vi "create_request_and_send.vi"(8 "error in":errorcluster, 11 "obj in":refnum<class "RequestBuilder.lvclass">) -> (0 "error out":errorcluster, 2 "request":refnum<class "Request.lvclass">, 3 "obj out":refnum<class "RequestBuilder.lvclass">)   [LabVIEW 2020, in "reqwest.lvlib" / "RequestBuilder.lvclass"]
uses:
  RequestBuilder.lvclass
  Request/Request.lvclass
  Request/request_id.ctl
  RequestBuilder.lvclass/RequestBuilder.ctl
  lv_reqwest_32.dll
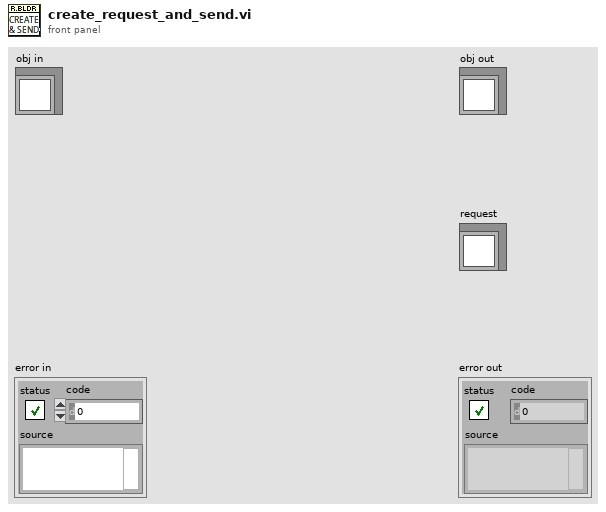
[diagram p1: front panel]
types:
  T1 = typedef "reqwest.lvlib/Request.lvclass/request_id.ctl" = u64
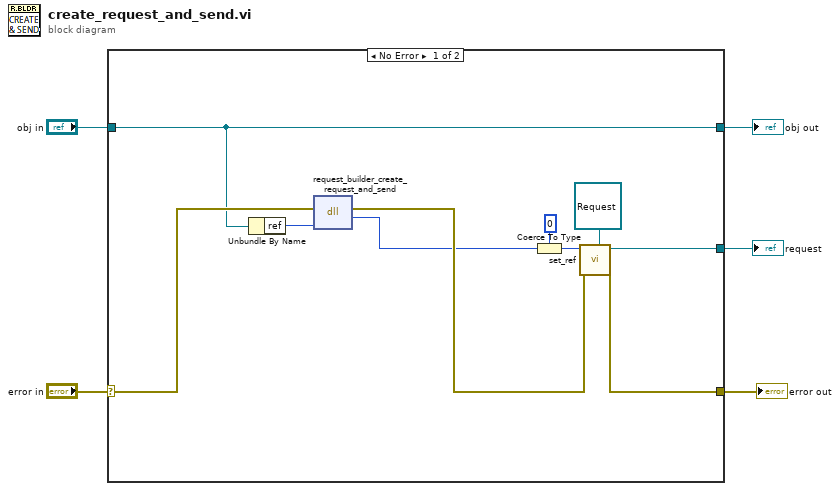
[diagram p0: block diagram]
diagram:
  n1 = case shown="No Error" "error in" {
    selector: "error in" -> [w15 w17]
    tunnel: "obj in" -> [w6 w16]
    tunnel: [w12 w17] -> w3
    tunnel: [w11 _] -> w2
    tunnel: [w6 w16] -> w1
    frame No Error {
      n2 = Unbundle By Name(w6) -> ("ref"=w14:u64)
      n3 = dll-call lib="C:/Projects/reqwest-rs-labview/lv_src/lv_reqwest_*.*" fn="request_builder_create_request_and_send"(error in=w15, "request_builder_ref"=w14) -> (error out=w13:errorcluster, "request_id"=w10:u64)  [unwired: 3 in, 1 out]
      n4 = Coerce To Type(0:w10, 1:T1 0 ("request_id")) -> (2:w8:T1)
      n5 = call "set_ref.vi"("Request in"=refnum<class "Request.lvclass"> refnum, "error in (no error)"=w13, "request_id"=w8) -> ("error out"=w12:errorcluster, "Request out"=w11:refnum<class "Request.lvclass">)  [unwired: 7 in]
    }
    frame Error {
    }
  }
  "error out" <- w3
  "request" <- w2
  "obj out" <- w1
